vi "Execute.vi"(8 "error in (no error)":errorcluster, 10 "Msg Queue":refnum<queue>, 11 "Message in":refnum<class "Message.lvclass">=refnum) -> (0 "error out":errorcluster, 3 "Message out":refnum<class "Message.lvclass">)   [LabVIEW 2020, in "State Machine.lvlib"]
uses:
  State Machine.lvlib
  OOP SM/Stop Msg/Stop Msg.lvclass
  OOP SM/Message/Message.lvclass
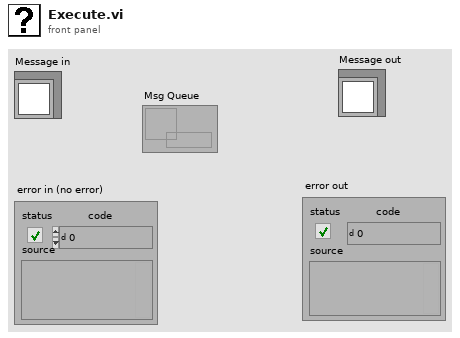
[diagram p1: front panel]
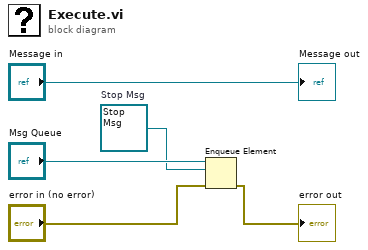
[diagram p0: block diagram]
diagram:
  w3 = refnum<class "Stop Msg.lvclass"> refnum  # Stop Msg
  n1 = Enqueue Element(queue="Msg Queue", element=w3, error in (no error)="error in (no error)") -> (error out=→"error out":errorcluster)  [unwired: 1 in, 2 out]
  "Message out" <- "Message in"
